vi "Sequence.Test.CreateDMC.vi"(5 "Default":bool, 6 "TS (now)":timestamp, 7 "GUI? (F)":bool, 8 "Serial (0)":i32, 9 "DMCConfig":T7, 10 "Plate":T1, 11 "Variant":T2={"State"=enum."Init", "ImgPath"=path "", "WabcoPlate"="", "WabcoProduct"="", "ClientProduct"="", "ClientPlate"="", "TotalQuantity"=0, "OrderQuantity"=0, "Serial"=0, "Wabco"={"LaserJob"="", "AdditionalTxt"="037", "FactoryCode"="", "RevID"=0, "ForkID"=0, "FailuresLimit"=0, "GlobalCnt"=0, "Bank"=0, "SerialFormat"=enum."6 dig", "CoordA"={"X"=0.0, "Y"=0.0, "Angle"=0.0}, "CoordB"={"X"=0.0, "Y"=0.0, "Angle"=0.0}, "DMCconfig"=0}, "Client"={"LaserJob"="", "AdditionalTxt"="", "FactoryCode"="037", "RevID"=0, "ForkID"=0, "FailuresLimit"=0, "GlobalCnt"=0, "Bank"=0, "SerialFormat"=enum."6 dig", "CoordA"={"X"=0.0, "Y"=0.0, "Angle"=0.0}, "CoordB"={"X"=0.0, "Y"=0.0, "Angle"=0.0}, "DMCconfig"=0}}) -> (1 "DMC nok":bool, 3 "DMC":string)   [LabVIEW 2016]
uses:
  Gui/DMCConfiguatorGui.ConfigData.ctl
  Gui/DMCConfiguatorGui.Component.ctl
  Gui/DMCConfiguatorGui.Type.ctl
  Gui/DMCConfiguatorGui.Var.ctl
  Logger/Logger.Variant.Sets.ctl
  Station/Station.Changeover.State.vi
  Station/Station.Plate.Properties.ctl
  Sequence.Code.SerialFormat.ctl
  Drivers/V7310/LowLevel/V7310.Job.Sets.ctl
  Sequence.PlateType.ctl
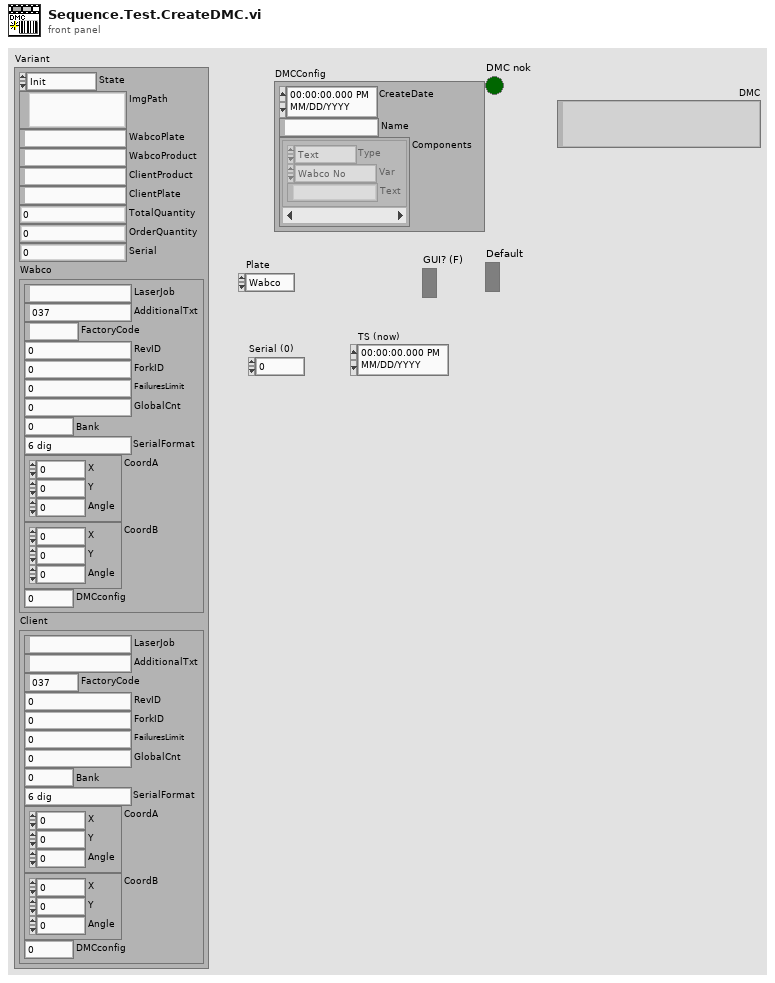
[diagram p1: front panel]
types:
  T1 = typedef "Sequence.PlateType.ctl" = enum16{"Wabco", "Client"}
  T2 = typedef "Logger.Variant.Sets.ctl" = cluster{"State":T3, "ImgPath":path, "WabcoPlate":string, "WabcoProduct":string, "ClientProduct":string, "ClientPlate":string, "TotalQuantity":u16, "OrderQuantity":u16, "Serial":i32, "Wabco":T4, "Client":T4}
  T3 = typedef "Station.Changeover.State.vi" = enum16{"Init", "Scaning", "NOK", "Wait for ack", "Ready"}
  T4 = typedef "Station.Plate.Properties.ctl" = cluster{"LaserJob":string, "AdditionalTxt":string, "FactoryCode":string, "RevID":u8, "ForkID":u8, "FailuresLimit":u16, "GlobalCnt":i32, "Bank":u8, "SerialFormat":T5, "CoordA":T6, "CoordB":T6, "DMCconfig":i32}
  T5 = typedef "Sequence.Code.SerialFormat.ctl" = enum8{"", "6 dig", "7 dig"}
  T6 = typedef "V7310.Job.Sets.ctl" = cluster{"X":dbl, "Y":dbl, "Angle":dbl}
  T7 = typedef "DMCConfiguatorGui.ConfigData.ctl" = cluster{"CreateDate":timestamp, "Name":string, "Components":T8[]}
  T8 = typedef "DMCConfiguatorGui.Component.ctl" = cluster{"Type":T9, "Var":T10, "Text":string}
  T9 = typedef "DMCConfiguatorGui.Type.ctl" = enum8{"Text", "Variable"}
  T10 = typedef "DMCConfiguatorGui.Var.ctl" = enum8{"-", "Wabco No", "Client No", "Serial", "Date"}
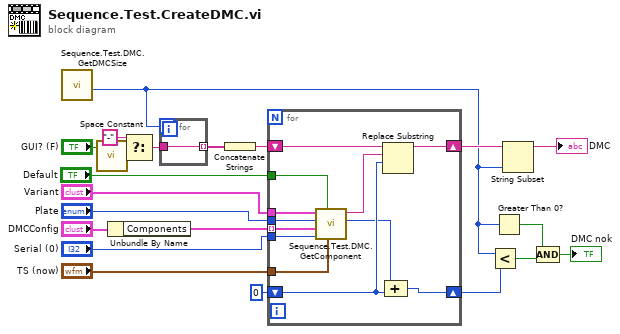
[diagram p0: block diagram]
diagram:
  n1 = call "Sequence.Test.DMC.GetDMCSize.vi"() -> ("max size"=w3:i32)  [unwired: 11 in]
  n2 = call <vilib>:"Space Constant.vi"() -> ("String"=w9:string)
  n3 = Unbundle By Name("DMCConfig") -> ("Components"=w15:T8[])
  n4 = Select(t="-", s="GUI? (F)", f=w9) -> (s? t:f=w7:string)
  n5 = for {
    N: w3 -> [_]
    tunnel: [w22] -> w21 mode=indexing
    tunnel: w7 -> [w22]
  }
  n6 = Concatenate Strings(w21) -> (w20:string)
  n7 = for {
    tunnel: w15 -> [w30] mode=indexing
    shift-right: [w33] -> w19
    shift-left: w20 -> [w34]
    shift-right: [w31] -> w5
    shift-left: 0 -> [w32]
    tunnel: "Plate" -> [w29]
    tunnel: "Variant" -> [w28]
    tunnel: "Serial (0)" -> [w27]
    tunnel: "TS (now)" -> [w24]
    tunnel: "Default" -> [w23]
    n8 = call "Sequence.Test.DMC.GetComponent.vi"("TS (now)"=w24, "Default"=w23, "Cnt (0)"=w27, "Component"=w30, "Plate"=w29, "OrderSets"=w28) -> ("size"=w25:i32, "Value"=w26:string)  [unwired: 3 in, 1 out]
    n9 = Replace Substring(3:w32, 4:w26, 5:w34) -> (1:w33:string)  [unwired: 1 in, 1 out]
    n10 = Compound Arithmetic op=ADD(w25, w32) -> (w31:i32)
  }
  n11 = Less?(x=w3, y=w5) -> (x < y?=w4:bool)
  n12 = Greater Than 0?(x=w3) -> (x > 0?=w1:bool)
  n13 = String Subset(string=w19, length (rest)=w3) -> (substring=→"DMC":string)  [unwired: 1 in]
  n14 = Compound Arithmetic op=AND(w1, w4) -> (→"DMC nok":bool)
